vi "Linearly Spaced Array 2012 NIVerified.vi"(8 "error in (no error)":errorcluster, 9 "Number of Samples":i32, 10 "Maximum":dbl, 11 "Minimum":dbl) -> (0 "error out":errorcluster, 3 "Array":dbl[](array[numeric]))   [LabVIEW 2020]
doc: "This subVI will create an evenly spaced array of elements equal to the Number of Samples between the Minimum and Maximum"
panel:
  # "Overview: Generate array with equally spaced array elements.\nRequirements: LabVIEW Full Development System\nInstructions:\n1- Enter the minimum value (start value)\n2- Enter the maximum value (end value)\n3- Enter the number of samples (number of elements)\n4- Run the VI"
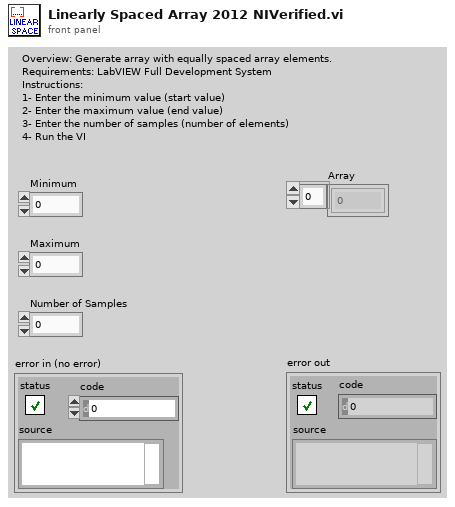
[diagram p1: front panel]
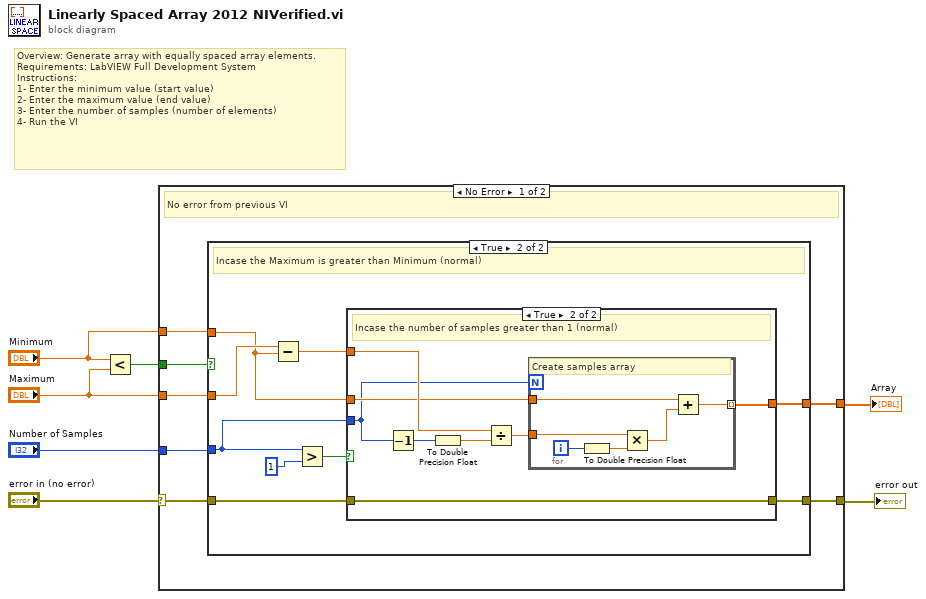
[diagram p0: block diagram]
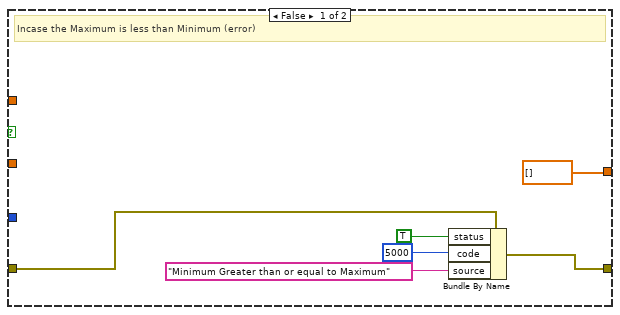
[diagram p2: hidden frame]
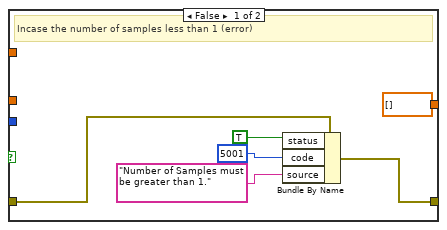
[diagram p3: hidden frame]
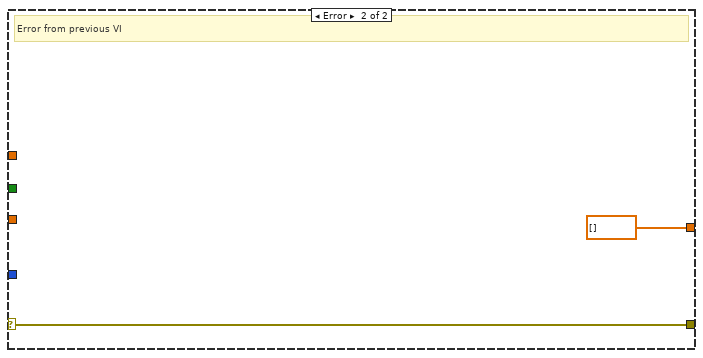
[diagram p4: hidden frame]
diagram:
  # "Overview: Generate array with equally spaced array elements.\nRequirements: LabVIEW Full Development System\nInstructions:\n1- Enter the minimum value (start value)\n2- Enter the maximum value (end value)\n3- Enter the number of samples (number of elements)\n4- Run the VI"
  n1 = Less?(x="Minimum", y="Maximum") -> (x < y?=w7:bool)
  n2 = case shown="No Error" "error in (no error)" {
    selector: "error in (no error)" -> [w9 w50]
    tunnel: w7 -> [w14 _]
    tunnel: "Maximum" -> [w13 _]
    tunnel: "Minimum" -> [w12 _]
    tunnel: [w11 w50] -> w6
    tunnel: "Number of Samples" -> [w10 _]
    tunnel: [w8 dbl[] []] -> w4
    frame No Error {
      # "No error from previous VI"
      n3 = case shown="True" w14 {
        tunnel: w9 -> [w20 w28]
        tunnel: [w16 w27] -> w11
        tunnel: w13 -> [_ w26]
        tunnel: w12 -> [_ w23]
        tunnel: w10 -> [_ w22]
        tunnel: [dbl[] [] w21] -> w8
        frame False {
          # "Incase the Maximum is less than Minimum (error)"
          n4 = Bundle By Name(cluster=w20, "status"=TRUE, "code"=5000, "source"="Minimum Greater than or equal to Maximum") -> (w16:errorcluster)
        }
        frame True {
          # "Incase the Maximum is greater than Minimum (normal)"
          n5 = Subtract(x=w26, y=w23) -> (x-y=w29:dbl)
          n6 = Greater?(x=w22, y=1) -> (0:w24:bool)
          n7 = case shown="True" w24 {
            tunnel: w29 -> [_ w43]
            tunnel: w28 -> [w35 w42]
            tunnel: [w34 w42] -> w27
            tunnel: w22 -> [_ w37]
            tunnel: w23 -> [_ w39]
            tunnel: [dbl[] [] w38] -> w21
            frame False {
              # "Incase the number of samples less than 1 (error)"
              n8 = Bundle By Name(cluster=w35, "status"=TRUE, "code"=5001, "source"="Number of Samples must be greater than 1.") -> (w34:errorcluster)
            }
            frame True {
              # "Incase the number of samples greater than 1 (normal)"
              n9 = Decrement(x=w37) -> (x-1=w41:i32)
              n10 = To Double Precision Float(number=w41) -> (double precision float=w36:dbl)
              n11 = Divide(x=w43, y=w36) -> (x/y=w40:dbl)
              n12 = for {
                N: w37 -> [_]
                tunnel: w39 -> [w45]
                tunnel: w40 -> [w48]
                tunnel: [w47] -> w38 mode=indexing
                i -> [w49]
                # "Create samples array"
                n13 = To Double Precision Float(number=w49) -> (double precision float=w46:dbl)
                n14 = Multiply(x=w48, y=w46) -> (x*y=w44:dbl)
                n15 = Add(x=w45, y=w44) -> (x+y=w47:dbl)
              }
            }
          }
        }
      }
    }
    frame Error {
      # "Error from previous VI"
    }
  }
  "error out" <- w6
  "Array" <- w4
